vi "Tabla.vi"() -> ()   [LabVIEW 2020]
panel:
  in  "stop":bool
  out "Table Control":string[][](table)
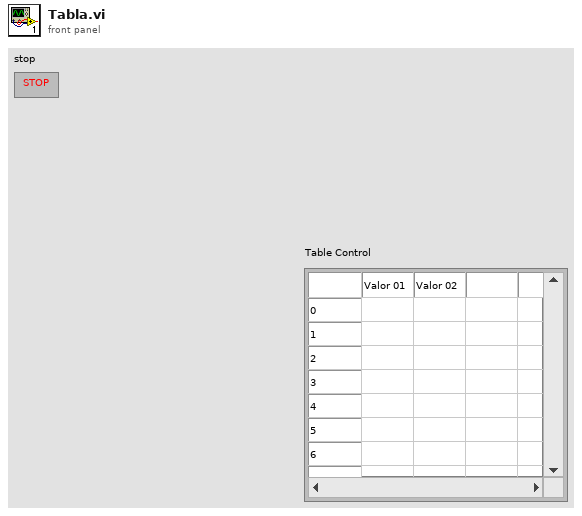
[diagram p1: front panel]
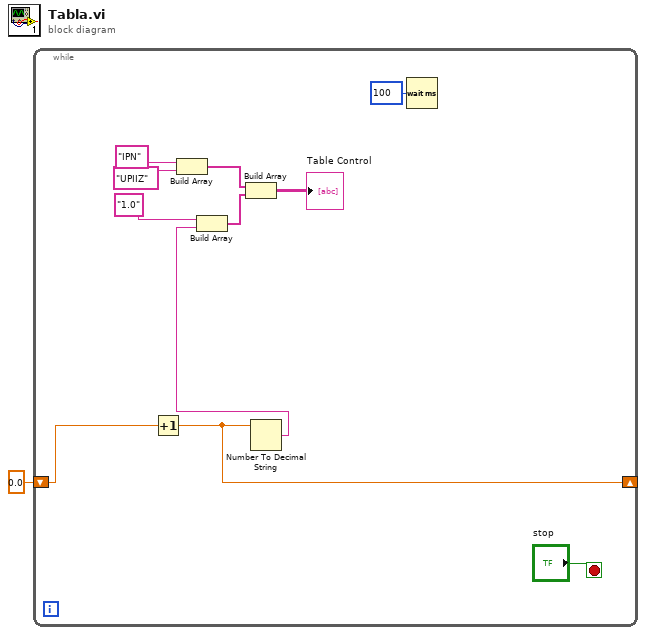
[diagram p0: block diagram]
diagram:
  n1 = while {
    shift-right: [w4] -> _
    shift-left: 0.0 -> [w3]
    stop <- "stop" stop-if-true
    n2 = Increment(x=w3) -> (x+1=w4:dbl)
    n3 = Build Array("IPN", "UPIIZ") -> (w11:string[])
    n4 = Number To Decimal String(number=w4) -> (decimal integer string=w2:string)  [unwired: 1 in]
    n5 = Build Array("1.0", w2) -> (w10:string[])
    n6 = Build Array(w11, w10) -> (→"Table Control":string[][])
    n7 = Wait (ms)(milliseconds to wait=u32 100) -> ()  [unwired: 1 out]
  }
